vi "Get SLSC Switch Resource.vi"(8 "error in (no error)":errorcluster, 11 "SLSC Sw Custom Device Ref in":T1 format="%.0x") -> (0 "error out":errorcluster, 2 "Resource":string, 3 "SLSC Sw Custom Device Ref out":T1 format="%.0x")   [LabVIEW 2017, in "SLSC Switch Scripting.lvlib"]
uses:
  SLSC Switch Scripting.lvlib
  <vilib>/NI Veristand/Custom Device API/Custom Device Item Ref.ctl
  SLSC Scripting Constants.vi
  <vilib>/NI Veristand/Custom Device API/Get Item Property (String).vi
  <vilib>/NI VeriStand/Custom Device API/Custom Device API.lvlib
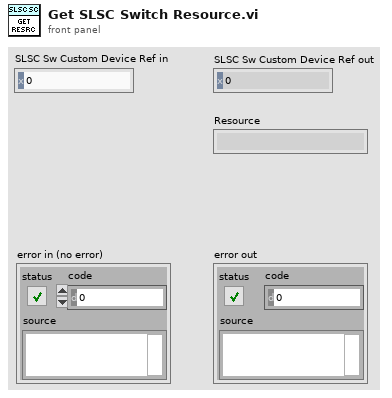
[diagram p1: front panel]
types:
  T1 = typedef "Custom Device API.lvlib/Custom Device Item Ref.ctl" = u64
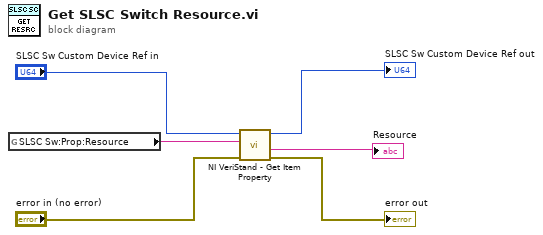
[diagram p0: block diagram]
diagram:
  n1 = global read "SLSC Scripting Constants.vi" "SLSC Sw:Prop:Resource"() -> (w3:string)
  n2 = call-poly <vilib>:"NI VeriStand - Get Item Property.vi"("error in (no error)"="error in (no error)", "Property Name"=w3, "Item Ref in"="SLSC Sw Custom Device Ref in") -> ("error out"=→"error out":errorcluster, "Value"=→"Resource":string, "Item Ref out"=→"SLSC Sw Custom Device Ref out":T1)  [unwired: 5 in, 1 out]
